vi "Object Detection SubVI.vi"(4 "Error In":errorcluster, 5 "Mode":enum16{"Ball", "Soap", "Gel", "Pipe", "None"}(ring), 6 "Image Dest":T1, 7 "Image in":T1) -> (0 "Error out":errorcluster, 1 "Object Center Coordinates":cluster{"x":sgl, "y":sgl}, 2 "Object detection cluster":T2, 3 "Image Out":T1)   [LabVIEW 2018]
uses:
  <vilib>/vision/Image Controls.llb/IMAQ Image.ctl
panel:
  out "Image":T1(plugin-control)
  out "Ball detected":bool
  out "Pipe detected":bool
  out "Gel detected":bool
  out "Soap detected":bool
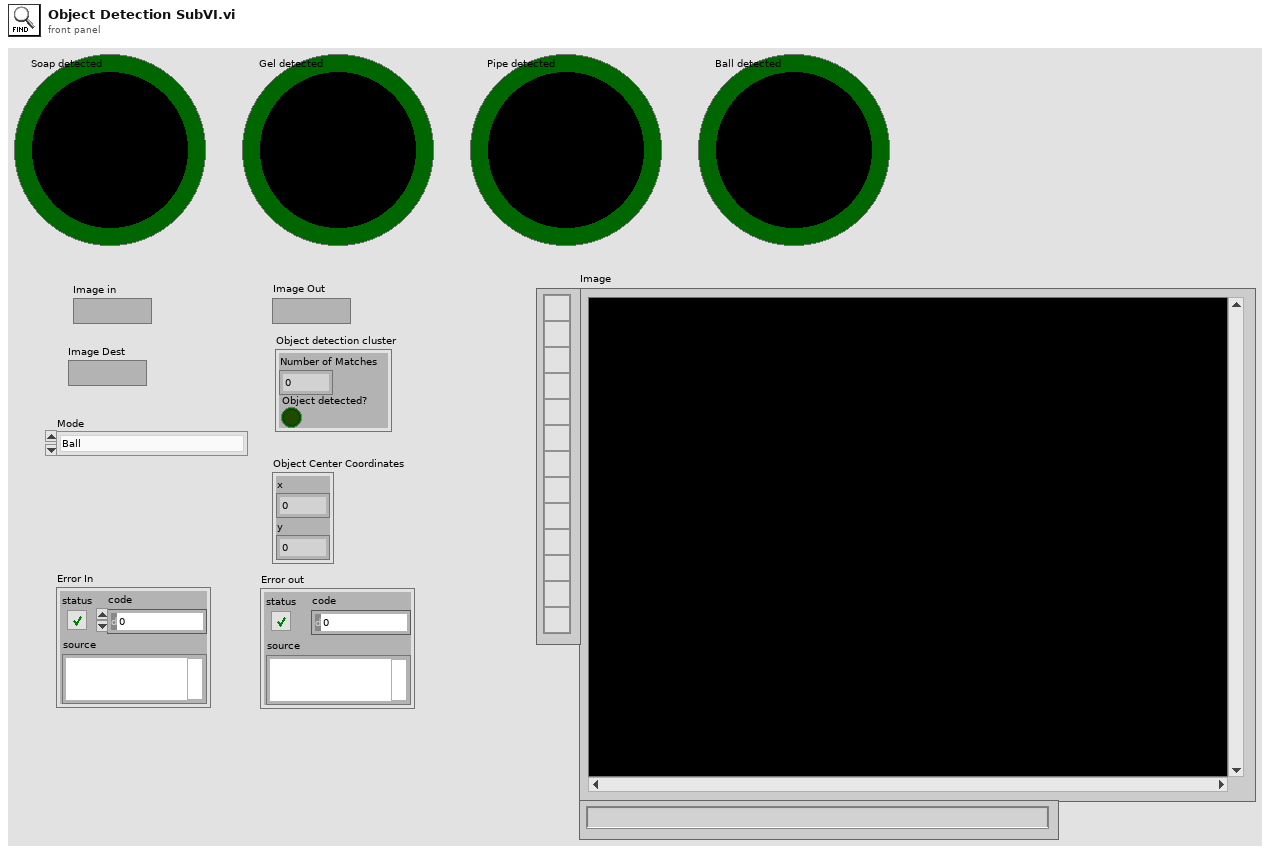
[diagram p1: front panel]
types:
  T1 = typedef "IMAQ Image.ctl" = refnum<image>
  T2 = cluster{"Number of Matches":i32, "Object detected?":bool}
  T3 = cluster{"Position":cluster{"x":sgl, "y":sgl}, "Angle":sgl, "Scale":sgl, "Score":sgl, "Bounding Box":cluster{"x":sgl, "y":sgl}[]}[]
  T4 = typedef "IMAQ GM Match Report.ctl" = cluster{"Position":cluster{"x":sgl, "y":sgl}, "Angle":sgl, "Scale":sgl, "Score":sgl, "Bounding Box":cluster{"x":sgl, "y":sgl}[], "Contrast Reversed":bool, "Occlusion %":sgl, "Template Target Curve Score":sgl, "Target Template Curve Score":sgl, "Correlation Score":sgl}
  T5 = cluster{"Calibrated Matches (Pattern Matching 1)[0]":T4, "Calibrated Matches (Pattern Matching 1)[1]":T4, "Calibrated Matches (Pattern Matching 1)[2]":T4, "Calibrated Matches (Pattern Matching 1)[3]":T4, "Calibrated Matches (Pattern Matching 1)[4]":T4, "Calibrated Matches (Pattern Matching 1)[5]":T4, "Calibrated Matches (Pattern Matching 1)[6]":T4, "Calibrated Matches (Pattern Matching 1)[7]":T4, "Calibrated Matches (Pattern Matching 1)[8]":T4}
  T6 = cluster{"Matches (calibrated) (Color Location 1)[0]":cluster{"Position":cluster{"x":sgl, "y":sgl}, "Angle":sgl, "Scale":sgl, "Score":sgl, "Bounding Box":cluster{"x":sgl, "y":sgl}[]}, "Matches (calibrated) (Color Location 1)[1]":cluster{"Position":cluster{"x":sgl, "y":sgl}, "Angle":sgl, "Scale":sgl, "Score":sgl, "Bounding Box":cluster{"x":sgl, "y":sgl}[]}, "Matches (calibrated) (Color Location 1)[2]":cluster{"Position":cluster{"x":sgl, "y":sgl}, "Angle":sgl, "Scale":sgl, "Score":sgl, "Bounding Box":cluster{"x":sgl, "y":sgl}[]}, "Matches (calibrated) (Color Location 1)[3]":cluster{"Position":cluster{"x":sgl, "y":sgl}, "Angle":sgl, "Scale":sgl, "Score":sgl, "Bounding Box":cluster{"x":sgl, "y":sgl}[]}, "Matches (calibrated) (Color Location 1)[4]":cluster{"Position":cluster{"x":sgl, "y":sgl}, "Angle":sgl, "Scale":sgl, "Score":sgl, "Bounding Box":cluster{"x":sgl, "y":sgl}[]}, "Matches (calibrated) (Color Location 1)[5]":cluster{"Position":cluster{"x":sgl, "y":sgl}, "Angle":sgl, "Scale":sgl, "Score":sgl, "Bounding Box":cluster{"x":sgl, "y":sgl}[]}, "Matches (calibrated) (Color Location 1)[6]":cluster{"Position":cluster{"x":sgl, "y":sgl}, "Angle":sgl, "Scale":sgl, "Score":sgl, "Bounding Box":cluster{"x":sgl, "y":sgl}[]}, "Matches (calibrated) (Color Location 1)[7]":cluster{"Position":cluster{"x":sgl, "y":sgl}, "Angle":sgl, "Scale":sgl, "Score":sgl, "Bounding Box":cluster{"x":sgl, "y":sgl}[]}, "Matches (calibrated) (Color Location 1)[8]":cluster{"Position":cluster{"x":sgl, "y":sgl}, "Angle":sgl, "Scale":sgl, "Score":sgl, "Bounding Box":cluster{"x":sgl, "y":sgl}[]}}
  T7 = cluster{"Position":cluster{"x":sgl, "y":sgl}, "Angle":sgl, "Scale":sgl, "Score":sgl, "Bounding Box":cluster{"x":sgl, "y":sgl}[]}
  T8 = cluster{"Number of Matches (Pattern Matching 1)":i32, bool}
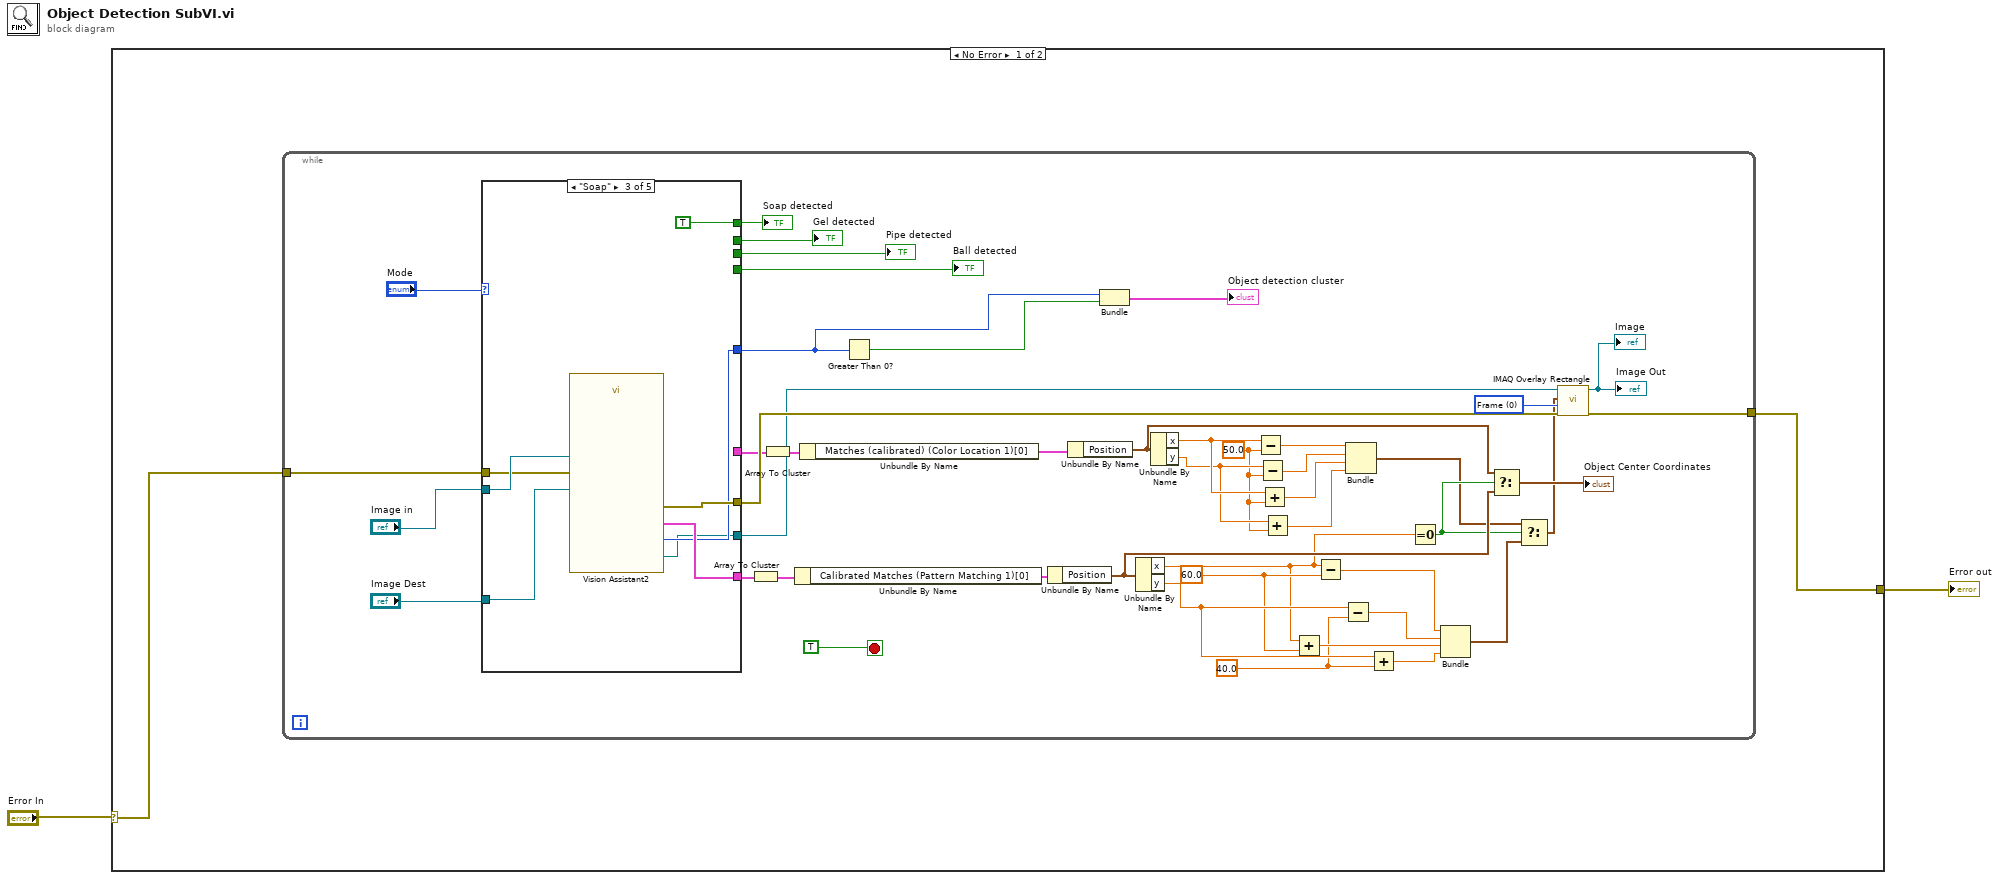
[diagram p0: block diagram]
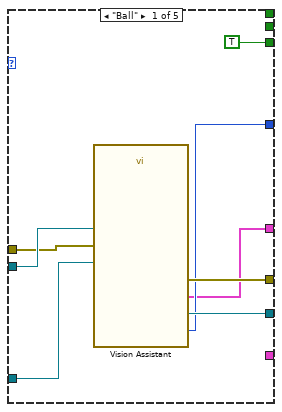
[diagram p2: hidden frame]
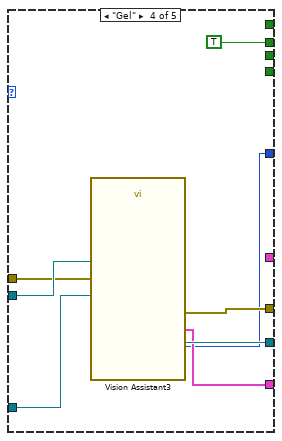
[diagram p4: hidden frame]
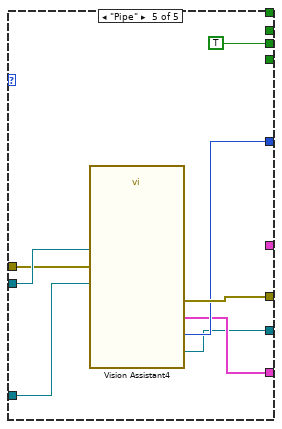
[diagram p5: hidden frame]
diagram:
  n1 = case shown="No Error" "Error In" {
    selector: "Error In" -> [w4 w84]
    tunnel: [w3 w84] -> w2
    frame No Error {
      n2 = while {
        tunnel: w4 -> [w33]
        tunnel: [w32] -> w3
        stop <- TRUE ("Stop (F)") stop-if-true
        w19 = sgl 50.0 ("y")
        w34 = sgl 60.0 ("y")
        w37 = sgl 40.0 ("y")
        w47 = u32 0 items=["Frame", "Fill", "Highlight"] ("Drawing Mode (Frame)")
        n3 = case shown="\"Soap\"" "Mode" {
          tunnel: [w57 w59 w67 w75 w83] -> w46
          tunnel: "Image in" -> [w56 w58 w66 w74 w82]
          tunnel: "Image Dest" -> [w55 _ w65 w73 w81]
          tunnel: [w51 _ w63 w68 w80] -> w27
          tunnel: [_ _ w64 w69 w79] -> w45
          tunnel: [w54 w58 w62 w72 w78] -> w35
          tunnel: w33 -> [w53 w59 w61 w71 w77]
          tunnel: [_ _ TRUE _ _] -> w31
          tunnel: [_ _ _ TRUE _] -> w30
          tunnel: [_ _ _ _ TRUE] -> w29
          tunnel: [TRUE _ _ _ _] -> w28
          tunnel: [w50 _ _ _ _] -> w8
          frame "Ball" {
            n4 = call "Vision Assistant"("Image In"=w56, "Image Dst"=w55, "error in"=w53) -> ("Image Out"=w54:T1, "Number of Matches (Color Location 1)"=w51:i32, "Matches (calibrated) (Color Location 1)"=w50:T3, "error out"=w57:errorcluster)  [unwired: 21 in]
          }
          frame "None", Default {
          }
          frame "Soap" {
            n5 = call "Vision Assistant2"("Image In"=w66, "Image Dst"=w65, "error in"=w61) -> ("Image Out"=w62:T1, "Number of Matches (Pattern Matching 1)"=w63:i32, "Calibrated Matches (Pattern Matching 1)"=w64:T4[], "error out"=w67:errorcluster)  [unwired: 21 in]
          }
          frame "Gel" {
            n6 = call "Vision Assistant3"("Image In"=w74, "Image Dst"=w73, "error in"=w71) -> ("Image Out"=w72:T1, "Calibrated Matches (Pattern Matching 1)"=w69:T4[], "Number of Matches (Pattern Matching 1)"=w68:i32, "error out"=w75:errorcluster)  [unwired: 21 in]
          }
          frame "Pipe" {
            n7 = call "Vision Assistant4"("Image In"=w82, "Image Dst"=w81, "error in"=w77) -> ("Image Out"=w78:T1, "Number of Matches (Pattern Matching 1)"=w80:i32, "Calibrated Matches (Pattern Matching 1)"=w79:T4[], "error out"=w83:errorcluster)  [unwired: 21 in]
          }
        }
        "Soap detected" <- w31
        "Pipe detected" <- w29
        "Ball detected" <- w28
        "Gel detected" <- w30
        n8 = Array To Cluster(array=w45) -> (cluster=w44:T5)
        n9 = Array To Cluster(array=w8) -> (cluster=w7:T6)
        n10 = Unbundle By Name(w44) -> ("Calibrated Matches (Pattern Matching 1)[0]"=w43:T4)
        n11 = Unbundle By Name(w7) -> ("Matches (calibrated) (Color Location 1)[0]"=w6:T7)
        n12 = Greater Than 0?(x=w27) -> (x > 0?=w26:bool)
        n13 = Unbundle By Name(w43) -> ("Position"=w15:cluster{"x":sgl, "y":sgl})
        n14 = Unbundle By Name(w6) -> ("Position"=w14:cluster{"x":sgl, "y":sgl})
        n15 = Bundle("Number of Matches (Pattern Matching 1)"=w27, w26) -> (→"Object detection cluster":T8)  [unwired: 1 in]
        n16 = Unbundle By Name(w15) -> ("x"=w13:sgl, "y"=w39:sgl)
        n17 = Unbundle By Name(w14) -> ("x"=w21:sgl, "y"=w20:sgl)
        n18 = Subtract(x=w21, y=w19) -> (x-y=w23:sgl)
        n19 = Subtract(x=w20, y=w19) -> (x-y=w22:sgl)
        n20 = Add(x=w21, y=w19) -> (x+y=w18:sgl)
        n21 = Add(x=w20, y=w19) -> (x+y=w17:sgl)
        n22 = Add(x=w13, y=w34) -> (x+y=w42:sgl)
        n23 = Subtract(x=w13, y=w34) -> (x-y=w40:sgl)
        n24 = Subtract(x=w39, y=w37) -> (x-y=w38:sgl)
        n25 = Bundle(w23, w22, w18, w17) -> (w10:cluster{sgl, sgl, sgl, sgl})  [unwired: 1 in]
        n26 = Add(x=w39, y=w37) -> (x+y=w41:sgl)
        n27 = Equal To 0?(x=w13) -> (x = 0?=w11:bool)
        n28 = Bundle(w40, w38, w42, w41) -> (w12:cluster{sgl, sgl, sgl, sgl})  [unwired: 1 in]
        n29 = Select(t=w14, s=w11, f=w15) -> (s? t:f=→"Object Center Coordinates":cluster{"x":sgl, "y":sgl})
        n30 = Select(t=w10, s=w11, f=w12) -> (s? t:f=w9:cluster{sgl, sgl, sgl, sgl})
        n31 = call "IMAQ Overlay Rectangle"("error in (no error)"=w46, "Drawing Mode (Frame)"=w47, "Rectangle"=w9, "Image"=w35) -> ("error out"=w32:errorcluster, "Image Out"=→"Image Out" →"Image":T1)  [unwired: 6 in]
      }
    }
    frame Error {
    }
  }
  "Error out" <- w2
